vi "rs3_close all2.vi"(6 "rscontext":u64, 7 "queue in":u64, 8 "error in (no error)":errorcluster, 9 "device_list":u64, 10 "Dev in":u64, 11 "Sensor in":u64) -> (0 "error out (no error)":errorcluster, 3 "Close Error":string)   [LabVIEW 2018, in "libRealSense3.lvlib"]
doc: "It is important to close everything properly at the end. Use this VI to clean up and close the RealSense device, queue, sensor, and device list."
uses:
  libRealSense3.lvlib
panel:
  # "RS3 Close All"
  # "(C) Intel Corp. 2017,  AGJ"
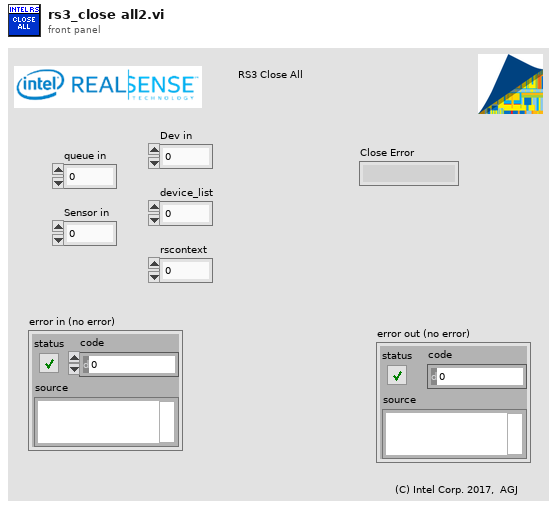
[diagram p1: front panel]
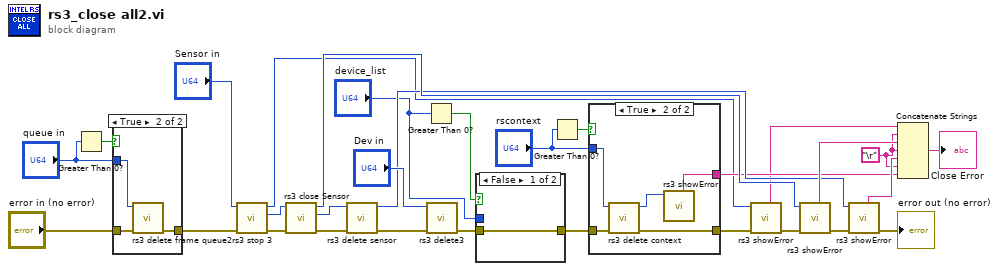
[diagram p0: block diagram]
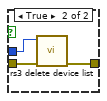
[diagram p2: hidden frame]
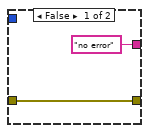
[diagram p4: hidden frame]
diagram:
  w13 = "\r"
  n1 = Greater Than 0?(x="queue in") -> (x > 0?=w9:bool)
  n2 = case shown="True" w9 {
    tunnel: "error in (no error)" -> [w31 w34]
    tunnel: "queue in" -> [_ w33]
    tunnel: [w31 w32] -> w17
    frame False {
    }
    frame True {
      n3 = call "rs3 delete frame queue2.vi"("error in (no error)"=w34, "queue"=w33) -> ("error out"=w32:errorcluster)  [unwired: 9 in]
    }
  }
  n4 = call "rs3 stop 3.vi"("error in (no error)"=w17, "sensor"="Sensor in") -> ("error out"=w16:errorcluster, "sensor out"=w14:u64, "error"=w11:u64)  [unwired: 7 in]
  n5 = call "rs3 close Sensor.vi"("error in (no error)"=w16, "sensor"=w14) -> ("error out"=w28:errorcluster, "device out"=w27:u64, "error"=w20:u64)  [unwired: 7 in]
  n6 = call "rs3 delete sensor.vi"("error in (no error)"=w28, "sensor"=w27) -> ("error out"=w29:errorcluster, "error"=w19:u64)  [unwired: 8 in]
  n7 = Greater Than 0?(x="device_list") -> (x > 0?=w1:bool)
  n8 = call "rs3 delete3.vi"("error in (no error)"=w29, "device"="Dev in") -> ("error out"=w24:errorcluster)  [unwired: 9 in]
  n9 = case shown="False" w1 {
    tunnel: [w35 w38] -> w26
    tunnel: w24 -> [w35 w37]
    tunnel: "device_list" -> [_ w36]
    frame False {
    }
    frame True {
      n10 = call "rs3 delete device list.vi"("error in (no error)"=w37, "device list"=w36) -> ("error out"=w38:errorcluster)  [unwired: 9 in]
    }
  }
  n11 = Greater Than 0?(x="rscontext") -> (x > 0?=w7:bool)
  n12 = case shown="True" w7 {
    tunnel: w26 -> [w39 w45]
    tunnel: [w39 w44] -> w6
    tunnel: ["no error" ("Error summary") w42] -> w18
    tunnel: "rscontext" -> [_ w41]
    frame False {
    }
    frame True {
      n13 = call "rs3 delete context.vi"("error in (no error)"=w45, "context"=w41) -> ("error out"=w44:errorcluster, "error"=w43:u64)  [unwired: 8 in]
      n14 = call "rs3 showError.vi"("error"=w43) -> ("Error summary"=w42:string)  [unwired: 6 in, 4 out]
    }
  }
  n15 = call "rs3 showError.vi"("error in (no error)"=w6, "error"=w11) -> ("error out"=w5:errorcluster, "Error summary"=w12:string)  [unwired: 5 in, 3 out]
  n16 = call "rs3 showError.vi"("error in (no error)"=w5, "error"=w20) -> ("error out"=w4:errorcluster, "Error summary"=w23:string)  [unwired: 5 in, 3 out]
  n17 = call "rs3 showError.vi"("error in (no error)"=w4, "error"=w19) -> ("error out"=→"error out (no error)":errorcluster, "Error summary"=w22:string)  [unwired: 5 in, 3 out]
  n18 = Concatenate Strings(w12, w13, w23, w13, w22, w13, w18) -> (→"Close Error":string)
